vi "Blink.vi"(8 "Error In":errorcluster) -> (0 "Error Out":errorcluster, 3 "concatenated string":string)   [LabVIEW 2014]
uses:
  Basic API/ctl/pinDirection.ctl
  Basic API/ctl/digitalPin.ctl
panel:
  in  "sketch name":string="__generated_LuboJ_out"
  out "standard error":string
  out "standard output":string
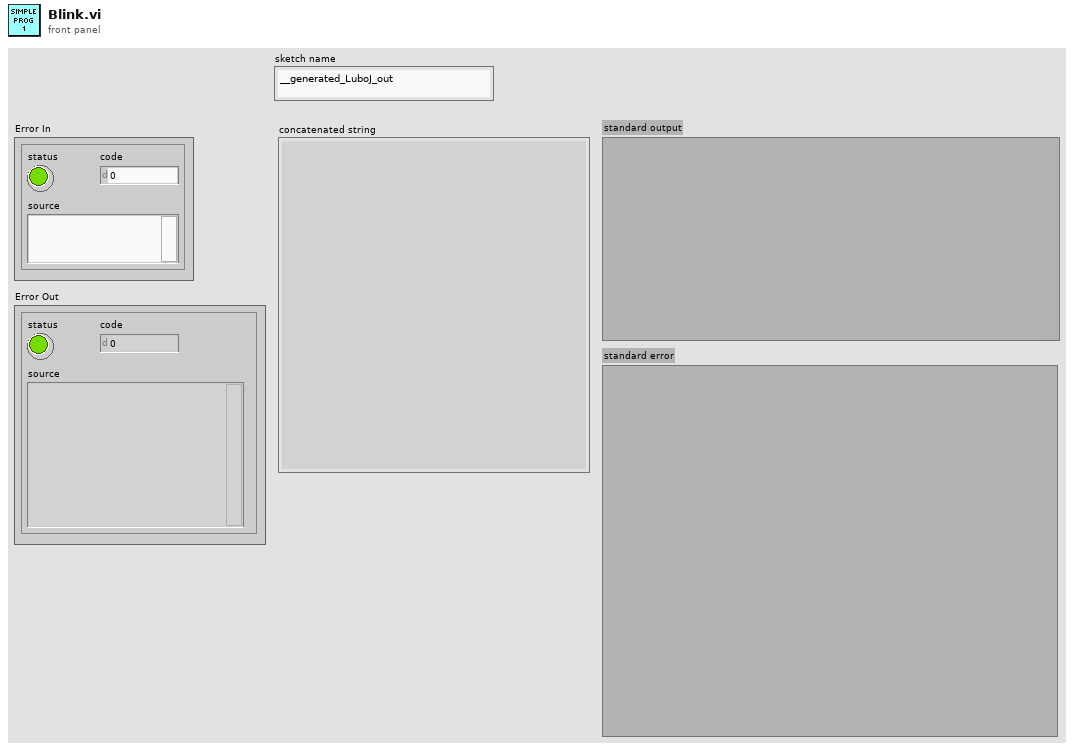
[diagram p1: front panel]
types:
  T1 = typedef "digitalPin.ctl" = u16
  T2 = typedef "pinDirection.ctl" = enum16{"INPUT", "OUTPUT"}
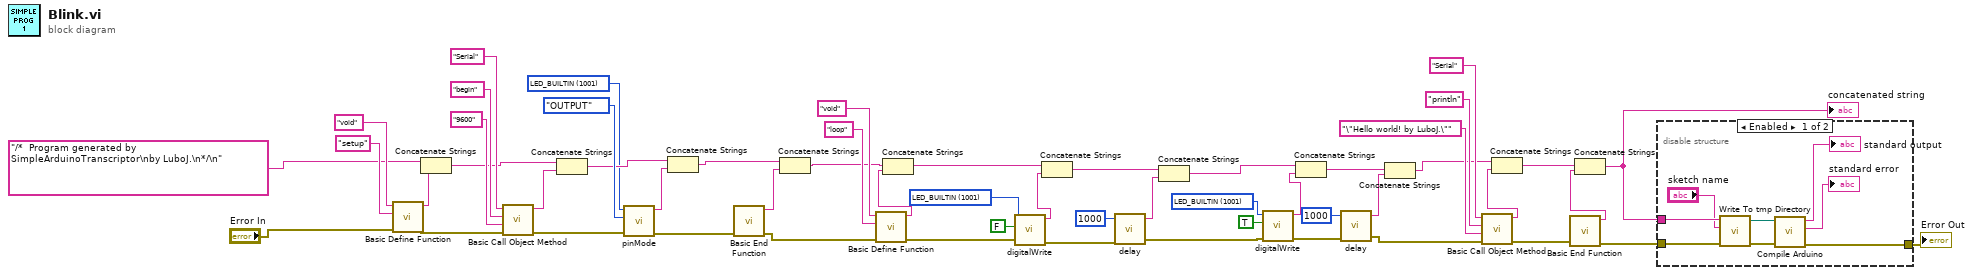
[diagram p0: block diagram]
diagram:
  w1 = T1 1001 items=["D0"=0, "D1"=1, "D2"=2, "D3"=3, "D4"=4, "D5"=5, "D6"=6, "D7"=7, "D8"=8, "D9"=9, "D10"=10, "D11"=11, "D12"=12, "D13"=13, "D14"=14, "D15"=15, "LED_BUILTIN"=1001] ("Digital Pin")
  w2 = T1 1001 items=["D0"=0, "D1"=1, "D2"=2, "D3"=3, "D4"=4, "D5"=5, "D6"=6, "D7"=7, "D8"=8, "D9"=9, "D10"=10, "D11"=11, "D12"=12, "D13"=13, "D14"=14, "D15"=15, "LED_BUILTIN"=1001] ("Digital Pin")
  w3 = T1 1001 items=["D0"=0, "D1"=1, "D2"=2, "D3"=3, "D4"=4, "D5"=5, "D6"=6, "D7"=7, "D8"=8, "D9"=9, "D10"=10, "D11"=11, "D12"=12, "D13"=13, "D14"=14, "D15"=15, "LED_BUILTIN"=1001] ("pin")
  n1 = call "Basic Define Function.vi"("Error In"="Error In", "name"="setup", "return type"="void") -> ("Error Out"=w47:errorcluster, "concatened string"=w52:string)  [unwired: 7 in]
  n2 = Concatenate Strings("/*  Program generated by SimpleArduinoTranscriptor\nby LuboJ.\n*/\n" ("string"), w52) -> (w43:string)
  n3 = call "Basic Call Object Method.vi"("Error In"=w47, "args"="9600", "method"="begin", "object name"="Serial") -> ("Error Out"=w9:errorcluster, "concatened string"=w44:string)  [unwired: 6 in]
  n4 = Concatenate Strings(w43, w44) -> (w6:string)
  n5 = call "pinMode.vi"("Error In"=w9, "Pin Direction"=pinDirection."OUTPUT", "pin"=w3) -> ("Error Out"=w7:errorcluster, "resulting string"=w5:string)  [unwired: 7 in]
  n6 = Concatenate Strings(w6, w5) -> (w4:string)
  n7 = call "Basic End Function.vi"("Error In"=w7) -> ("Error Out"=w31:errorcluster, "resulting string"=w51:string)  [unwired: 9 in]
  n8 = Concatenate Strings(w4, w51) -> (w38:string)
  n9 = call "Basic Define Function.vi"("Error In"=w31, "name"="loop", "return type"="void") -> ("Error Out"=w27:errorcluster, "concatened string"=w40:string)  [unwired: 7 in]
  n10 = Concatenate Strings(w38, w40) -> (w25:string)
  n11 = call "digitalWrite.vi"("Error In"=w27, "value"=FALSE, "Digital Pin"=w2) -> ("Error Out"=w23:errorcluster, "resulting string"=w26:string)  [unwired: 7 in]
  n12 = Concatenate Strings(w25, w26) -> (w20:string)
  n13 = call "delay.vi"("Error In"=w23, "time (ms)"=u32 1000) -> ("Error Out"=w18:errorcluster, "resulting string"=w21:string)  [unwired: 2 in]
  n14 = Concatenate Strings(w20, w21) -> (w13:string)
  n15 = call "digitalWrite.vi"("Error In"=w18, "value"=TRUE, "Digital Pin"=w1) -> ("Error Out"=w15:errorcluster, "resulting string"=w14:string)  [unwired: 7 in]
  n16 = Concatenate Strings(w13, w14) -> (w12:string)
  n17 = call "delay.vi"("Error In"=w15, "time (ms)"=u32 1000) -> ("Error Out"=w10:errorcluster, "resulting string"=w17:string)  [unwired: 2 in]
  n18 = Concatenate Strings(w12, w17) -> (w11:string)
  n19 = call "Basic Call Object Method.vi"("Error In"=w10, "args"="\"Hello world! by LuboJ.\"", "method"="println", "object name"="Serial") -> ("Error Out"=w32:errorcluster, "concatened string"=w34:string)  [unwired: 6 in]
  n20 = Concatenate Strings(w11, w34) -> (w33:string)
  n21 = call "Basic End Function.vi"("Error In"=w32) -> ("Error Out"=w30:errorcluster, "resulting string"=w39:string)  [unwired: 9 in]
  n22 = Concatenate Strings(w33, w39) -> (w29:string)
  "concatenated string" <- w29
  n23 = disable-structure shown="Enabled" {
    disable-tunnel: w30 -> [w62 w63]
    disable-tunnel: w29 -> [w61 _]
    disable-tunnel: [w58 w63] -> w28
    frame Enabled {
      n24 = call "Write To tmp Directory.vi"("error in (no error)"=w62, "sketch name"="sketch name", "arduino code"=w61) -> ("error out"=w60:errorcluster, "output file"=w59:path)  [unwired: 7 in]
      n25 = call "Compile Arduino.vi"("Error In"=w60, "input filename"=w59) -> ("Error Out"=w58:errorcluster, "standard error"=→"standard error":string, "standard output"=→"standard output":string)  [unwired: 7 in]
    }
    frame Disabled {
    }
  }
  "Error Out" <- w28
